vi "AOL Properties - Reorder.vi"(7 "Function":T1, 9 "Value":T2={"AOD 1 thickness (mm)"=8.0, "AOD 2 thickness (mm)"=8.0, "AOD 3 thickness (mm)"=8.0, "AOD 4 thickness (mm)"=8.0, "AOD 1-2 separation (mm)"=50.0, "AOD 2-3 separation (mm)"=50.0, "AOD 3-4 separation (mm)"=50.0, "AOD 1 Centre (mm)"=7.5, "AOD 2 Centre (mm)"=7.5, "AOD 3 Centre (mm)"=7.5, "AOD 4 Centre (mm)"=7.5, "AOD 1 X Offset"=0.0, "AOD 2 X Offset"=0.0023, "AOD 3 X Offset"=0.0046, "AOD 4 X Offset"=0.0046, "AOD 1 Y Offset"=0.0, "AOD 2 Y Offset"=0.0, "AOD 3 Y Offset"=0.0023, "AOD 4 Y Offset"=0.0046, "Timing Offset AOD 1"=0.0, "Timing Offset AOD 2"=0.0, "Timing Offset AOD 3"=0.0, "Timing Offset AOD 4"=0.0, "AOL centre wavelength (nm)"=1.0, "AOL centre frequency (MHz)"=1.0, "Pair deflection ratio"=1.0, "AOL aperture (mm)"=15.0, "AOD fill time (us)"=1.0, "Diffraction mode"=1.0, "Crystal length (mm)"=0.0, "Acoustic velocity (m/s)"=1.0, "AOD Ord. Refractive index"=2.22}, 10 "AOL Properties out":T3={"AOD 1 thickness (mm)"=8.0, "AOD 2 thickness (mm)"=8.0, "AOD 3 thickness (mm)"=8.0, "AOD 4 thickness (mm)"=8.0, "AOD 5 thickness (mm)"=8.0, "AOD 6 thickness (mm)"=8.0, "AOD 1-2 separation (mm)"=50.0, "AOD 2-3 separation (mm)"=50.0, "AOD 3-4 separation (mm)"=50.0, "AOD 4-5 separation (mm)"=50.0, "AOD 5-6 separation (mm)"=50.0, "AOD 1 X Offset"=0.0, "AOD 2 X Offset"=0.0023, "AOD 3 X Offset"=0.0046, "AOD 4 X Offset"=0.0046, "AOD 1 Y Offset"=0.0, "AOD 2 Y Offset"=0.0, "AOD 3 Y Offset"=0.0023, "AOD 4 Y Offset"=0.0046, "AOD 1 X Direction"=0.0, "AOD 2 X Direction"=0.0, "AOD 3 X Direction"=0.0, "AOD 4 X Direction"=0.0, "AOD 1 Y Direction"=1.0, "AOD 2 Y Direction"=0.0, "AOD 3 Y Direction"=0.0023, "AOD 4 Y Direction"=0.0046, "AOD 1 Centre (mm)"=7.5, "AOD 2 Centre (mm)"=7.5, "AOD 3 Centre (mm)"=7.5, "AOD 4 Centre (mm)"=7.5, "Timing Offset AOD 1"=0.0, "Timing Offset AOD 2"=0.0, "Timing Offset AOD 3"=0.0, "Timing Offset AOD 4"=0.0, "AOD Optical offset 1"=20000.0, "AOD Optical offset 2"=20000.0, "AOL aperture (mm)"=15.0, "AOL centre wavelength (nm)"=1.0, "AOL centre frequency (MHz)"=1.0, "Diffraction mode"=1.0, "Crystal length (mm)"=0.0, "Acoustic velocity (m/s)"=1.0, "Pair deflection ratio"=1.0, "AOD fill time (us)"=1.0, "AOD Ord. Refractive index"=2.22, "AOD ExtraOrd. Refractive index"=2.22}) -> (1 "AOL Properties out":T3={"AOD 1 thickness (mm)"=8.0, "AOD 2 thickness (mm)"=8.0, "AOD 3 thickness (mm)"=8.0, "AOD 4 thickness (mm)"=8.0, "AOD 5 thickness (mm)"=8.0, "AOD 6 thickness (mm)"=8.0, "AOD 1-2 separation (mm)"=50.0, "AOD 2-3 separation (mm)"=50.0, "AOD 3-4 separation (mm)"=50.0, "AOD 4-5 separation (mm)"=50.0, "AOD 5-6 separation (mm)"=50.0, "AOD 1 X Offset"=0.0, "AOD 2 X Offset"=0.0023, "AOD 3 X Offset"=0.0046, "AOD 4 X Offset"=0.0046, "AOD 1 Y Offset"=0.0, "AOD 2 Y Offset"=0.0, "AOD 3 Y Offset"=0.0023, "AOD 4 Y Offset"=0.0046, "AOD 1 X Direction"=0.0, "AOD 2 X Direction"=0.0, "AOD 3 X Direction"=0.0, "AOD 4 X Direction"=0.0, "AOD 1 Y Direction"=1.0, "AOD 2 Y Direction"=0.0, "AOD 3 Y Direction"=0.0023, "AOD 4 Y Direction"=0.0046, "AOD 1 Centre (mm)"=7.5, "AOD 2 Centre (mm)"=7.5, "AOD 3 Centre (mm)"=7.5, "AOD 4 Centre (mm)"=7.5, "Timing Offset AOD 1"=0.0, "Timing Offset AOD 2"=0.0, "Timing Offset AOD 3"=0.0, "Timing Offset AOD 4"=0.0, "AOD Optical offset 1"=20000.0, "AOD Optical offset 2"=20000.0, "AOL aperture (mm)"=15.0, "AOL centre wavelength (nm)"=1.0, "AOL centre frequency (MHz)"=1.0, "Diffraction mode"=1.0, "Crystal length (mm)"=0.0, "Acoustic velocity (m/s)"=1.0, "Pair deflection ratio"=1.0, "AOD fill time (us)"=1.0, "AOD Ord. Refractive index"=2.22, "AOD ExtraOrd. Refractive index"=2.22}, 2 "Value":T2={"AOD 1 thickness (mm)"=8.0, "AOD 2 thickness (mm)"=8.0, "AOD 3 thickness (mm)"=8.0, "AOD 4 thickness (mm)"=8.0, "AOD 1-2 separation (mm)"=50.0, "AOD 2-3 separation (mm)"=50.0, "AOD 3-4 separation (mm)"=50.0, "AOD 1 Centre (mm)"=7.5, "AOD 2 Centre (mm)"=7.5, "AOD 3 Centre (mm)"=7.5, "AOD 4 Centre (mm)"=7.5, "AOD 1 X Offset"=0.0, "AOD 2 X Offset"=0.0023, "AOD 3 X Offset"=0.0046, "AOD 4 X Offset"=0.0046, "AOD 1 Y Offset"=0.0, "AOD 2 Y Offset"=0.0, "AOD 3 Y Offset"=0.0023, "AOD 4 Y Offset"=0.0046, "Timing Offset AOD 1"=0.0, "Timing Offset AOD 2"=0.0, "Timing Offset AOD 3"=0.0, "Timing Offset AOD 4"=0.0, "AOL centre wavelength (nm)"=1.0, "AOL centre frequency (MHz)"=1.0, "Pair deflection ratio"=1.0, "AOL aperture (mm)"=15.0, "AOD fill time (us)"=1.0, "Diffraction mode"=1.0, "Crystal length (mm)"=0.0, "Acoustic velocity (m/s)"=1.0, "AOD Ord. Refractive index"=2.22})   [LabVIEW 2020]
uses:
  Typedefs/AOD Settings-distilled.ctl
  Typedefs/AOL Properties Cluster.ctl
  User Interface/Visualisation/Functional Imaging Viewer/Typedefs/Get-Set-Clear Control.ctl
panel:
  # "Thickness (mm)"
  # "X Offset"
  # "Separation (mm)"
  # "Y Offset"
  # "Centre (mm)"
  # "Timing Offset"
  # "Thickness (mm)"
  # "X Offset"
  # "Separation (mm)"
  # "Y Offset"
  # "Centre (mm)"
  # "Timing Offset"
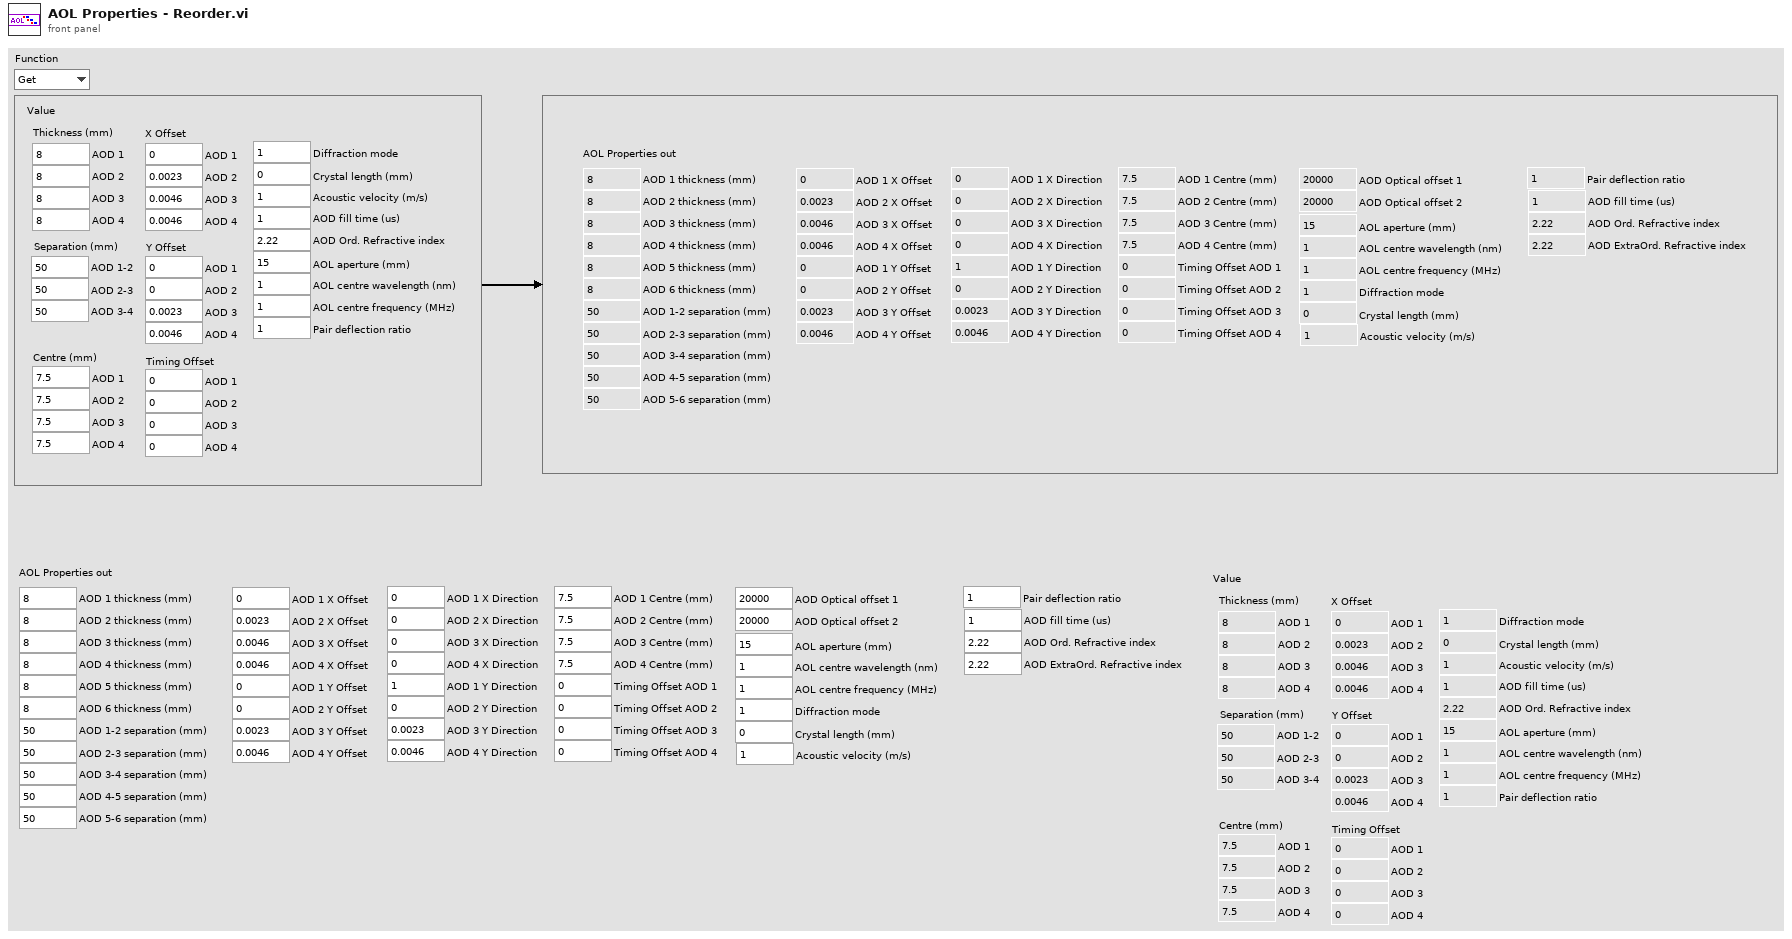
[diagram p1: front panel]
types:
  T1 = typedef "Get-Set-Clear Control.ctl" = enum16{"Get", "Set", "Clear"}
  T2 = typedef "AOD Settings-distilled.ctl" = cluster{"AOD 1 thickness (mm)":dbl, "AOD 2 thickness (mm)":dbl, "AOD 3 thickness (mm)":dbl, "AOD 4 thickness (mm)":dbl, "AOD 1-2 separation (mm)":dbl, "AOD 2-3 separation (mm)":dbl, "AOD 3-4 separation (mm)":dbl, "AOD 1 Centre (mm)":dbl, "AOD 2 Centre (mm)":dbl, "AOD 3 Centre (mm)":dbl, "AOD 4 Centre (mm)":dbl, "AOD 1 X Offset":dbl, "AOD 2 X Offset":dbl, "AOD 3 X Offset":dbl, "AOD 4 X Offset":dbl, "AOD 1 Y Offset":dbl, "AOD 2 Y Offset":dbl, "AOD 3 Y Offset":dbl, "AOD 4 Y Offset":dbl, "Timing Offset AOD 1":dbl, "Timing Offset AOD 2":dbl, "Timing Offset AOD 3":dbl, "Timing Offset AOD 4":dbl, "AOL centre wavelength (nm)":dbl, "AOL centre frequency (MHz)":dbl, "Pair deflection ratio":dbl, "AOL aperture (mm)":dbl, "AOD fill time (us)":dbl, "Diffraction mode":dbl, "Crystal length (mm)":dbl, "Acoustic velocity (m/s)":dbl, "AOD Ord. Refractive index":dbl}
  T3 = typedef "AOL Properties Cluster.ctl" = cluster{"AOD 1 thickness (mm)":dbl, "AOD 2 thickness (mm)":dbl, "AOD 3 thickness (mm)":dbl, "AOD 4 thickness (mm)":dbl, "AOD 5 thickness (mm)":dbl, "AOD 6 thickness (mm)":dbl, "AOD 1-2 separation (mm)":dbl, "AOD 2-3 separation (mm)":dbl, "AOD 3-4 separation (mm)":dbl, "AOD 4-5 separation (mm)":dbl, "AOD 5-6 separation (mm)":dbl, "AOD 1 X Offset":dbl, "AOD 2 X Offset":dbl, "AOD 3 X Offset":dbl, "AOD 4 X Offset":dbl, "AOD 1 Y Offset":dbl, "AOD 2 Y Offset":dbl, "AOD 3 Y Offset":dbl, "AOD 4 Y Offset":dbl, "AOD 1 X Direction":dbl, "AOD 2 X Direction":dbl, "AOD 3 X Direction":dbl, "AOD 4 X Direction":dbl, "AOD 1 Y Direction":dbl, "AOD 2 Y Direction":dbl, "AOD 3 Y Direction":dbl, "AOD 4 Y Direction":dbl, "AOD 1 Centre (mm)":dbl, "AOD 2 Centre (mm)":dbl, "AOD 3 Centre (mm)":dbl, "AOD 4 Centre (mm)":dbl, "Timing Offset AOD 1":dbl, "Timing Offset AOD 2":dbl, "Timing Offset AOD 3":dbl, "Timing Offset AOD 4":dbl, "AOD Optical offset 1":dbl, "AOD Optical offset 2":dbl, "AOL aperture (mm)":dbl, "AOL centre wavelength (nm)":dbl, "AOL centre frequency (MHz)":dbl, "Diffraction mode":dbl, "Crystal length (mm)":dbl, "Acoustic velocity (m/s)":dbl, "Pair deflection ratio":dbl, "AOD fill time (us)":dbl, "AOD Ord. Refractive index":dbl, "AOD ExtraOrd. Refractive index":dbl}
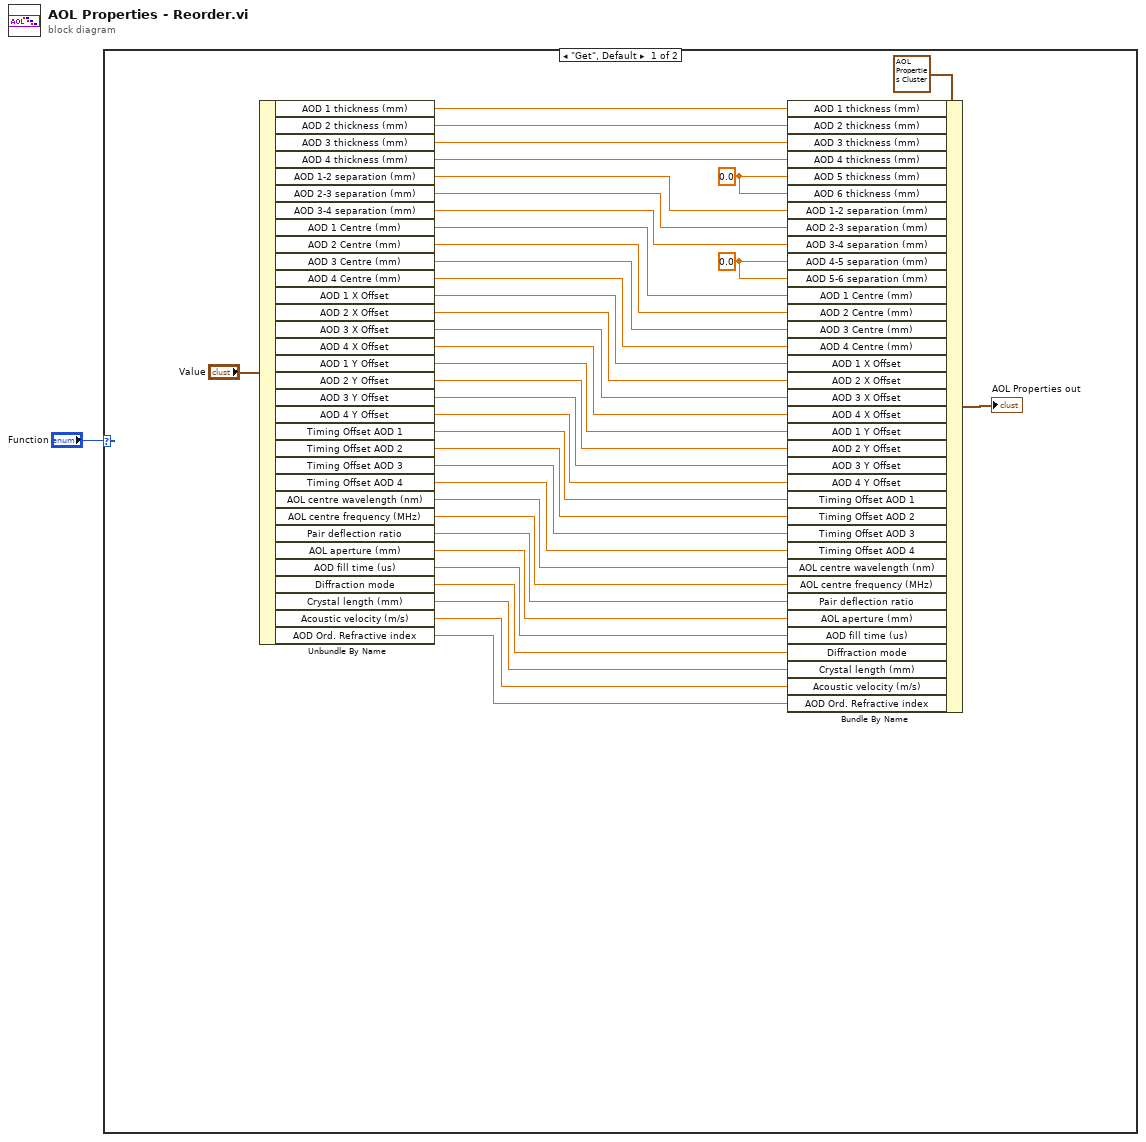
[diagram p0: block diagram]
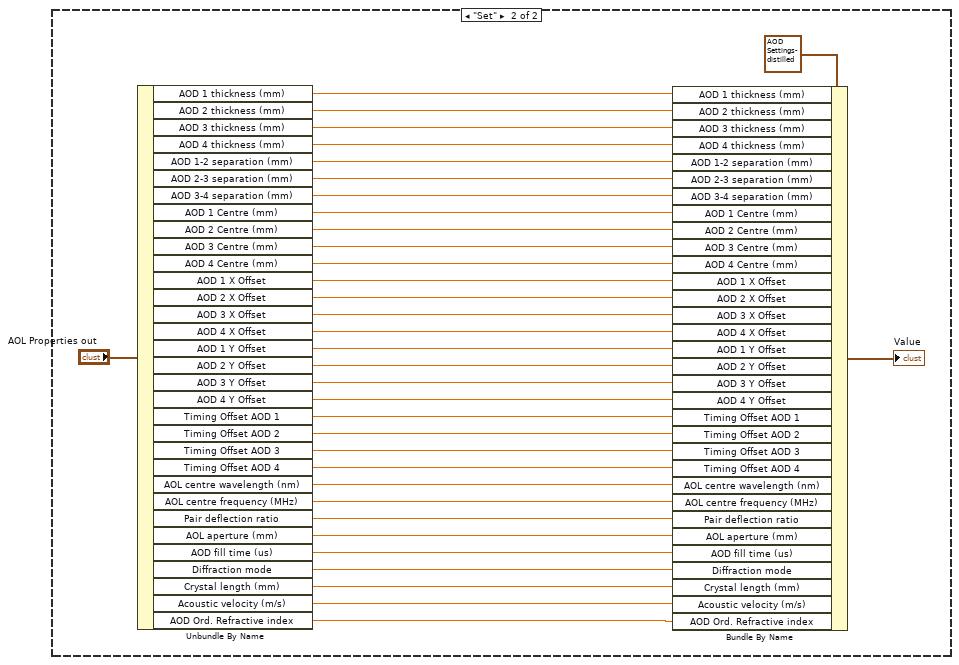
[diagram p2: hidden frame]
diagram:
  n1 = case shown="\"Get\", Default" "Function" {
    frame "Get", Default {
      w28 = 0.0 ("AOD 4-5 separation (mm)")
      w32 = 0.0 ("AOD 5 thickness (mm)")
      n2 = Unbundle By Name("Value") -> ("AOD 1 thickness (mm)"=w36:dbl, "AOD 2 thickness (mm)"=w35:dbl, "AOD 3 thickness (mm)"=w34:dbl, "AOD 4 thickness (mm)"=w33:dbl, "AOD 1-2 separation (mm)"=w31:dbl, "AOD 2-3 separation (mm)"=w30:dbl, "AOD 3-4 separation (mm)"=w29:dbl, "AOD 1 Centre (mm)"=w27:dbl, "AOD 2 Centre (mm)"=w26:dbl, "AOD 3 Centre (mm)"=w25:dbl, "AOD 4 Centre (mm)"=w24:dbl, "AOD 1 X Offset"=w23:dbl, "AOD 2 X Offset"=w22:dbl, "AOD 3 X Offset"=w21:dbl, "AOD 4 X Offset"=w20:dbl, "AOD 1 Y Offset"=w19:dbl, "AOD 2 Y Offset"=w18:dbl, "AOD 3 Y Offset"=w17:dbl, "AOD 4 Y Offset"=w16:dbl, "Timing Offset AOD 1"=w15:dbl, "Timing Offset AOD 2"=w14:dbl, "Timing Offset AOD 3"=w13:dbl, "Timing Offset AOD 4"=w12:dbl, "AOL centre wavelength (nm)"=w11:dbl, "AOL centre frequency (MHz)"=w10:dbl, "Pair deflection ratio"=w9:dbl, "AOL aperture (mm)"=w8:dbl, "AOD fill time (us)"=w7:dbl, "Diffraction mode"=w6:dbl, "Crystal length (mm)"=w5:dbl, "Acoustic velocity (m/s)"=w4:dbl, "AOD Ord. Refractive index"=w3:dbl)
      n3 = Bundle By Name(cluster=T3 {"AOD 1 thickness (mm)"=8.0, "AOD 2 thickness (mm)"=8.0, "AOD 3 thickness (mm)"=8.0, "AOD 4 thickness (mm)"=8.0, "AOD 5 thickness (mm)"=8.0, "AOD 6 thickness (mm)"=8.0, "AOD 1-2 separation (mm)"=50.0, "AOD 2-3 separation (mm)"=50.0, "AOD 3-4 separation (mm)"=50.0, "AOD 4-5 separation (mm)"=50.0, "AOD 5-6 separation (mm)"=50.0, "AOD 1 X Offset"=0.0, "AOD 2 X Offset"=0.0023, "AOD 3 X Offset"=0.0046, "AOD 4 X Offset"=0.0046, "AOD 1 Y Offset"=0.0, "AOD 2 Y Offset"=0.0, "AOD 3 Y Offset"=0.0023, "AOD 4 Y Offset"=0.0046, "AOD 1 X Direction"=0.0, "AOD 2 X Direction"=0.0, "AOD 3 X Direction"=0.0, "AOD 4 X Direction"=0.0, "AOD 1 Y Direction"=1.0, "AOD 2 Y Direction"=0.0, "AOD 3 Y Direction"=0.0023, "AOD 4 Y Direction"=0.0046, "AOD 1 Centre (mm)"=7.5, "AOD 2 Centre (mm)"=7.5, "AOD 3 Centre (mm)"=7.5, "AOD 4 Centre (mm)"=7.5, "Timing Offset AOD 1"=0.0, "Timing Offset AOD 2"=0.0, "Timing Offset AOD 3"=0.0, "Timing Offset AOD 4"=0.0, "AOD Optical offset 1"=20000.0, "AOD Optical offset 2"=20000.0, "AOL aperture (mm)"=15.0, "AOL centre wavelength (nm)"=1.0, "AOL centre frequency (MHz)"=1.0, "Diffraction mode"=1.0, "Crystal length (mm)"=0.0, "Acoustic velocity (m/s)"=1.0, "Pair deflection ratio"=1.0, "AOD fill time (us)"=1.0, "AOD Ord. Refractive index"=2.22, "AOD ExtraOrd. Refractive index"=2.22} ("AOL Properties"), "AOD 1 thickness (mm)"=w36, "AOD 2 thickness (mm)"=w35, "AOD 3 thickness (mm)"=w34, "AOD 4 thickness (mm)"=w33, "AOD 5 thickness (mm)"=w32, "AOD 6 thickness (mm)"=w32, "AOD 1-2 separation (mm)"=w31, "AOD 2-3 separation (mm)"=w30, "AOD 3-4 separation (mm)"=w29, "AOD 4-5 separation (mm)"=w28, "AOD 5-6 separation (mm)"=w28, "AOD 1 Centre (mm)"=w27, "AOD 2 Centre (mm)"=w26, "AOD 3 Centre (mm)"=w25, "AOD 4 Centre (mm)"=w24, "AOD 1 X Offset"=w23, "AOD 2 X Offset"=w22, "AOD 3 X Offset"=w21, "AOD 4 X Offset"=w20, "AOD 1 Y Offset"=w19, "AOD 2 Y Offset"=w18, "AOD 3 Y Offset"=w17, "AOD 4 Y Offset"=w16, "Timing Offset AOD 1"=w15, "Timing Offset AOD 2"=w14, "Timing Offset AOD 3"=w13, "Timing Offset AOD 4"=w12, "AOL centre wavelength (nm)"=w11, "AOL centre frequency (MHz)"=w10, "Pair deflection ratio"=w9, "AOL aperture (mm)"=w8, "AOD fill time (us)"=w7, "Diffraction mode"=w6, "Crystal length (mm)"=w5, "Acoustic velocity (m/s)"=w4, "AOD Ord. Refractive index"=w3) -> (→"AOL Properties out":T3)
    }
    frame "Set" {
      n4 = Unbundle By Name("AOL Properties out") -> ("AOD 1 thickness (mm)"=w71:dbl, "AOD 2 thickness (mm)"=w70:dbl, "AOD 3 thickness (mm)"=w69:dbl, "AOD 4 thickness (mm)"=w68:dbl, "AOD 1-2 separation (mm)"=w67:dbl, "AOD 2-3 separation (mm)"=w66:dbl, "AOD 3-4 separation (mm)"=w65:dbl, "AOD 1 Centre (mm)"=w64:dbl, "AOD 2 Centre (mm)"=w63:dbl, "AOD 3 Centre (mm)"=w62:dbl, "AOD 4 Centre (mm)"=w61:dbl, "AOD 1 X Offset"=w60:dbl, "AOD 2 X Offset"=w59:dbl, "AOD 3 X Offset"=w58:dbl, "AOD 4 X Offset"=w57:dbl, "AOD 1 Y Offset"=w56:dbl, "AOD 2 Y Offset"=w55:dbl, "AOD 3 Y Offset"=w54:dbl, "AOD 4 Y Offset"=w53:dbl, "Timing Offset AOD 1"=w52:dbl, "Timing Offset AOD 2"=w51:dbl, "Timing Offset AOD 3"=w50:dbl, "Timing Offset AOD 4"=w49:dbl, "AOL centre wavelength (nm)"=w48:dbl, "AOL centre frequency (MHz)"=w47:dbl, "Pair deflection ratio"=w46:dbl, "AOL aperture (mm)"=w45:dbl, "AOD fill time (us)"=w44:dbl, "Diffraction mode"=w43:dbl, "Crystal length (mm)"=w42:dbl, "Acoustic velocity (m/s)"=w41:dbl, "AOD Ord. Refractive index"=w40:dbl)
      n5 = Bundle By Name(cluster=T2 {"AOD 1 thickness (mm)"=8.0, "AOD 2 thickness (mm)"=8.0, "AOD 3 thickness (mm)"=8.0, "AOD 4 thickness (mm)"=8.0, "AOD 1-2 separation (mm)"=50.0, "AOD 2-3 separation (mm)"=50.0, "AOD 3-4 separation (mm)"=50.0, "AOD 1 Centre (mm)"=7.5, "AOD 2 Centre (mm)"=7.5, "AOD 3 Centre (mm)"=7.5, "AOD 4 Centre (mm)"=7.5, "AOD 1 X Offset"=0.0, "AOD 2 X Offset"=0.0023, "AOD 3 X Offset"=0.0046, "AOD 4 X Offset"=0.0046, "AOD 1 Y Offset"=0.0, "AOD 2 Y Offset"=0.0, "AOD 3 Y Offset"=0.0023, "AOD 4 Y Offset"=0.0046, "Timing Offset AOD 1"=0.0, "Timing Offset AOD 2"=0.0, "Timing Offset AOD 3"=0.0, "Timing Offset AOD 4"=0.0, "AOL centre wavelength (nm)"=1.0, "AOL centre frequency (MHz)"=1.0, "Pair deflection ratio"=1.0, "AOL aperture (mm)"=15.0, "AOD fill time (us)"=1.0, "Diffraction mode"=1.0, "Crystal length (mm)"=0.0, "Acoustic velocity (m/s)"=1.0, "AOD Ord. Refractive index"=2.22} ("Value"), "AOD 1 thickness (mm)"=w71, "AOD 2 thickness (mm)"=w70, "AOD 3 thickness (mm)"=w69, "AOD 4 thickness (mm)"=w68, "AOD 1-2 separation (mm)"=w67, "AOD 2-3 separation (mm)"=w66, "AOD 3-4 separation (mm)"=w65, "AOD 1 Centre (mm)"=w64, "AOD 2 Centre (mm)"=w63, "AOD 3 Centre (mm)"=w62, "AOD 4 Centre (mm)"=w61, "AOD 1 X Offset"=w60, "AOD 2 X Offset"=w59, "AOD 3 X Offset"=w58, "AOD 4 X Offset"=w57, "AOD 1 Y Offset"=w56, "AOD 2 Y Offset"=w55, "AOD 3 Y Offset"=w54, "AOD 4 Y Offset"=w53, "Timing Offset AOD 1"=w52, "Timing Offset AOD 2"=w51, "Timing Offset AOD 3"=w50, "Timing Offset AOD 4"=w49, "AOL centre wavelength (nm)"=w48, "AOL centre frequency (MHz)"=w47, "Pair deflection ratio"=w46, "AOL aperture (mm)"=w45, "AOD fill time (us)"=w44, "Diffraction mode"=w43, "Crystal length (mm)"=w42, "Acoustic velocity (m/s)"=w41, "AOD Ord. Refractive index"=w40) -> (→"Value":T2)
    }
  }
